vi "SVT Peak Sound Level (1 Ch).vi"(6 "restart averaging (F)":bool, 8 "error in (no error)":errorcluster, 11 "scaled signal [EU]":waveform(dbl)) -> (0 "error out":errorcluster, 2 "unit label":string, 3 "peak sound level [dB EU]":dbl=nan format="%.2f")   [LabVIEW 2017]
doc: "Computes <B>peak sound level [dB EU]</B> of <B>scaled signal [EU]</B>. You can use this polymorphic VI to compute the peak sound level for a single channel or for N channels. The data type you wire to the <B>scaled signal [EU]</B> input determines the polymorphic instance to use."
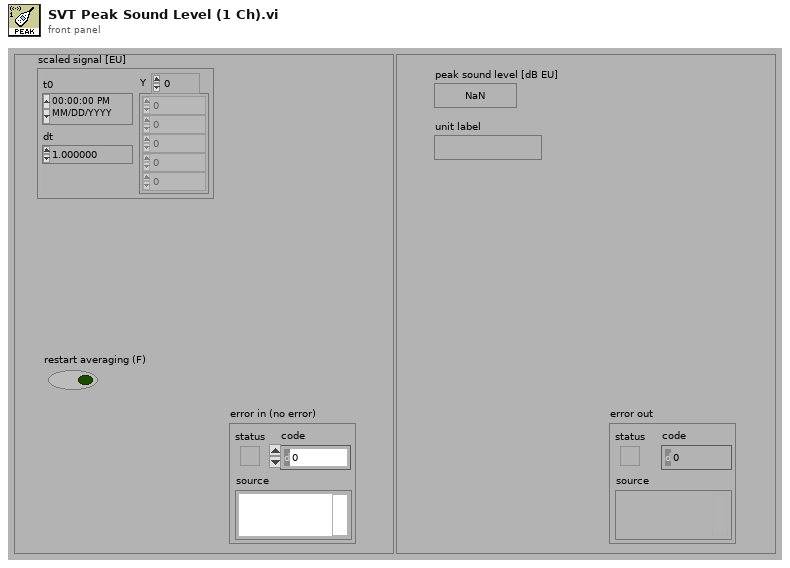
[diagram p1: front panel]
types:
  T1 = enum16{"RMS", "Running RMS", "Exp avg  ", "Dec exp avg ", "Peak", "Crest"}
  T2 = enum16{"Reset filter", "Restart averaging", "Continue processing"}
  T3 = typedef "svc_Channel Info.ctl" = cluster{"sensor sensitivity":dbl, "engineering units":T4, "dB reference":dbl, "custom label":string, "weighting filter":T5, "pregain":dbl}
  T4 = typedef "svc_Engineering Units Text Ring.ctl" = u16
  T5 = typedef "svc_Weighting Filter Text Ring.ctl" = u16
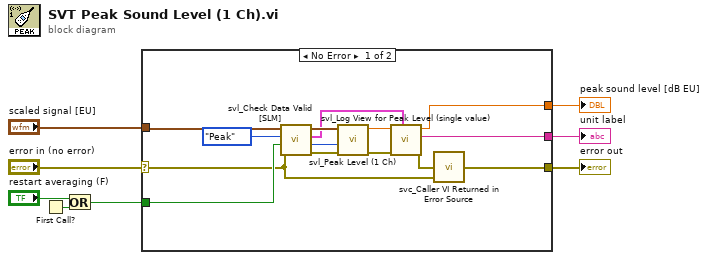
[diagram p0: block diagram]
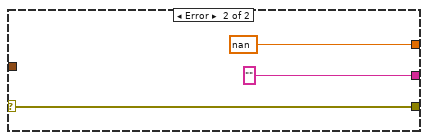
[diagram p2: hidden frame]
diagram:
  n1 = First Call?() -> (First Call?: T/F=w4:bool)
  n2 = Or(x="restart averaging (F)", y=w4) -> (x .or. y?=w2:bool)
  n3 = case shown="No Error" "error in (no error)" {
    selector: "error in (no error)" -> [w9 w25]
    tunnel: [w22 nan ("energy level [EU^2 rms]")] -> w8
    tunnel: [w21 "" ("unit label")] -> w7
    tunnel: [w17 w25] -> w6
    tunnel: "scaled signal [EU]" -> [w10 _]
    tunnel: w2 -> [w15 _]
    frame No Error {
      n4 = call <vilib>:"svl_Check Data Valid [SLM].vi"("error in (no error)"=w9, "restart averaging (F)"=w15, "Level Analysis"=T1."Peak", "scaled signal [EU]"=w10) -> ("error out"=w16:errorcluster, "processing state"=w14:T2, "channel info"=w11:T3, "dup scaled signal [EU]"=w12:waveform(dbl))  [unwired: 4 in]
      n5 = call <vilib>:"svl_Peak Level (1 Ch).vi"("error in (no error)"=w16, "processing state"=w14, "scaled signal"=w12) -> ("error out"=w19:errorcluster, "peak level"=w18:dbl)  [unwired: 7 in]
      n6 = call <vilib>:"svl_Log View for Peak Level (single value).vi"("channel info"=w11, "error in (no error)"=w19, "peak level [EU]"=w18) -> ("error out"=w20:errorcluster, "unit label"=w21:string, "peak level [EU]"=w22:dbl)  [unwired: 6 in]
      n7 = call <vilib>:"svc_Caller VI Returned in Error Source.vi"("warning input to caller"=w9, "error in (no error)"=w20) -> ("error out"=w17:errorcluster)  [unwired: 3 in]
    }
    frame Error {
    }
  }
  "peak sound level [dB EU]" <- w8
  "unit label" <- w7
  "error out" <- w6
